vi "GetGCSTranslatorDLLPath.vi"(1 "DLL Path (Required for Application, \nmust be set once for the application)":path) -> (0 "DLL path":path)   [LabVIEW 2020]
doc: "VI to create and store the path of the dynamic link libary GCSTranslator.dll (Windows) for the different bitnesses as function variable."
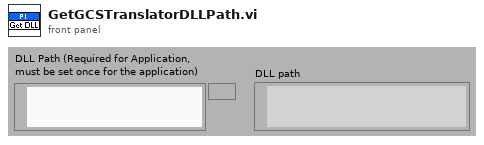
[diagram p1: front panel]
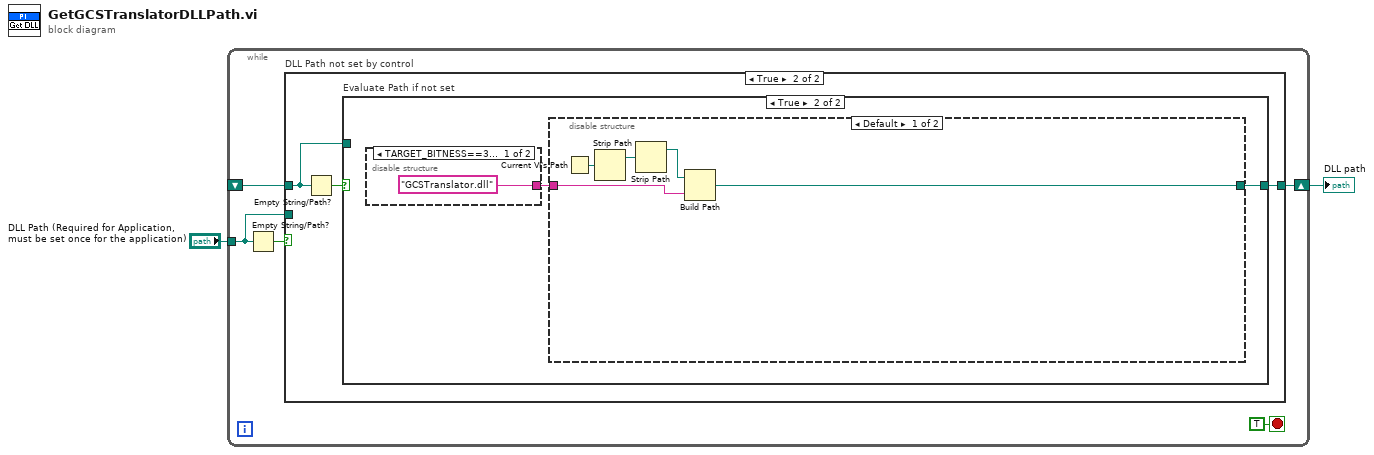
[diagram p0: block diagram]
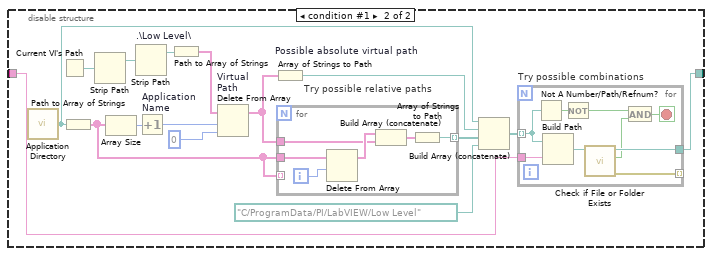
[diagram p4: hidden frame]
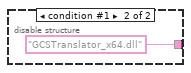
[diagram p5: hidden frame]
diagram:
  n1 = while {
    shift-right: [w7] -> w2
    shift-left: _ -> [w5]
    tunnel: "DLL Path (Required for Application, \nmust be set once for the application)" -> [w3]
    stop <- TRUE stop-if-true
    n2 = Empty String/Path?(string/path=w3) -> (empty?=w4:bool)
    n3 = case "DLL Path not set by control" shown="True" w4 {
      tunnel: [w8 w11] -> w7
      tunnel: w5 -> [_ w9]
      tunnel: w3 -> [w8 _]
      frame False {
      }
      frame True {
        n4 = Empty String/Path?(string/path=w9) -> (empty?=w10:bool)
        n5 = case "Evaluate Path if not set" shown="True" w10 {
          tunnel: [w12 w13] -> w11
          tunnel: w9 -> [w12 _]
          frame False {
          }
          frame True {
            n6 = disable-structure shown="TARGET_BITNESS==32" {
              disable-tunnel: ["GCSTranslator.dll" "GCSTranslator_x64.dll"] -> w14
              frame condition #0 (active) {
              }
              frame condition #1 {
              }
            }
            n7 = disable-structure shown="Default" {
              disable-tunnel: w14 -> [w19 w27]
              disable-tunnel: [w15 w28] -> w13
              frame condition #0 (active) {
                n8 = Current VI's Path() -> (path=w16:path)
                n9 = Strip Path(path=w16) -> (stripped path=w17:path)  [unwired: 1 out]
                n10 = Strip Path(path=w17) -> (stripped path=w18:path)  [unwired: 1 out]
                n11 = Build Path(base path=w18, name or relative path=w19) -> (appended path=w15:path)
              }
              frame condition #1 {
                n12 = call "Application Directory.vi"() -> ("Application Directory"=w24:path)
                n13 = Current VI's Path() -> (path=w30:path)
                n14 = Path to Array of Strings(0:w24) -> (2:w26:string[])  [unwired: 1 out]
                n15 = Strip Path(path=w30) -> (stripped path=w29:path)  [unwired: 1 out]
                n16 = Array Size(array=w26) -> (size(s)=w32:i32)
                n17 = Strip Path ".\\Low Level\\"(path=w29) -> (stripped path=w31:path)  [unwired: 1 out]
                n18 = Increment "Application\nName"(x=w32) -> (x+1=w34:i32)
                n19 = Path to Array of Strings(0:w31) -> (2:w35:string[])  [unwired: 1 out]
                n20 = Delete From Array "Virtual\nPath"(array=w35, length=w34, index=0) -> (array with subset deleted=w25:string[])  [unwired: 1 out]
                n21 = Array of Strings to Path "Possible absolute virtual path"(0:w25) -> (2:w23:path)  [unwired: 1 in]
                n22 = for "Try possible relative paths" {
                  tunnel: w26 -> [w47]
                  tunnel: w25 -> [w48]
                  tunnel: w26 -> [_] mode=indexing
                  tunnel: [w45] -> w21 mode=indexing
                  i -> [w50]
                  n23 = Delete From Array(array=w47, length=w50) -> (array with subset deleted=w49:string[])  [unwired: 1 in, 1 out]
                  n24 = Build Array (concatenate)(w49, w48) -> (w46:string[])
                  n25 = Array of Strings to Path(0:w46) -> (2:w45:path)  [unwired: 1 in]
                }
                n26 = Build Array (concatenate)(w24, w23, w21, path "C:/ProgramData/PI/LabVIEW/Low Level") -> (w20:path[])
                n27 = for "Try possible combinations" {
                  tunnel: [w44] -> w28
                  tunnel: w27 -> [w43]
                  tunnel: w20 -> [w41] mode=indexing
                  tunnel: [w36] -> _ mode=indexing
                  stop <- w37 stop-if-true
                  n28 = Not A Number/Path/Refnum?(number/path/refnum=w41) -> (NaN/Path/Refnum?=w40:bool)
                  n29 = Build Path(base path=w41, name or relative path=w43) -> (appended path=w42:path)
                  n30 = Not(x=w40) -> (.not. x?=w39:bool)
                  n31 = call "Check if File or Folder Exists.vi"("path"=w42) -> ("error out"=w36:errorcluster, "file or folder exists?"=w38:bool, "dup path"=w44:path)  [unwired: 8 in]
                  n32 = And(x=w39, y=w38) -> (x .and. y?=w37:bool)
                }
              }
            }
          }
        }
      }
    }
  }
  "DLL path" <- w2
